vi "PH_gentec_M-Link.set Wavelength.vi"(0 "i ref in":refnum<vi>, 2 "VISA resource in":refnum<visa-resource-name>, 5 "error in":errorcluster) -> (11 "Timeout":bool, 13 "Data read":string[](array[string]), 14 "i ref out":refnum<vi>, 16 "VISA resource out":refnum<visa-resource-name>, 17 "Error":bool, 18 "Failure":bool, 19 "error out":errorcluster)   [LabVIEW 2014, in "PH_gentec_M-Link.lvlib"]
doc: "This VI writes wanted Settings to the Device and checks the result."
uses:
  PH_gentec_M-Link.lvlib
  instr.lib/Gentec-M-Link/gentec-M-Link - Driver.lvlib
  PH_Basics/PH_Powermeter_BaseClass/PH_Powermeter_BaseClass.lvlib
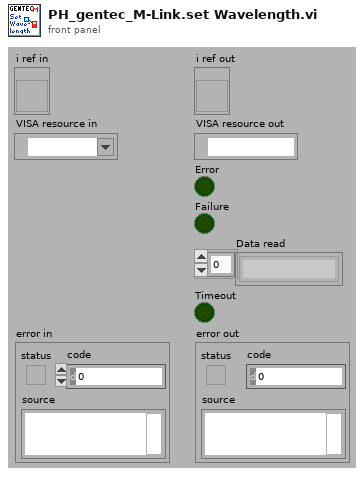
[diagram p1: front panel]
types:
  T1 = typedef "PH_Powermeter_BaseClass.lvlib/PH_Powermeter_BaseClass.i attribute.ctl" = cluster{"GUI References":T2, "Connection":T3, "Head Attributes":T5, "VISA resource":refnum<visa-resource-name>, "Energy":T6, "Service ID Energy":i32, "Wanted Settings":T7, "Current Settings":T7}
  T2 = typedef "PH_Powermeter_BaseClass.lvlib/PH_Powermeter_BaseClass.GUI Refs.ctl" = cluster{"Head Attributes":refnum<vi>, "Energy":refnum<vi>, "Connection":refnum<vi>, "VISA Resource":refnum<vi>, "Scaling Factor":refnum<vi>, "Range":refnum<vi>, "Wavelength":refnum<vi>, "Trigger Level":refnum<vi>, "Wanted Settings":refnum<vi>, "Current Settings":refnum<vi>}
  T3 = typedef "PH_Powermeter_BaseClass.lvlib/PH_Powermeter_BaseClass.Connection.ctl" = cluster{"failed checks":i8, "Timeout":bool, "Data read":string, "Failure":bool, "Error":bool, "State":T4}
  T4 = typedef "PH_Powermeter_BaseClass.lvlib/PH_Powermeter_BaseClass.State.ctl" = enum32{"off", "operating", "opened", "checked", "connected", "Sets to change", "running"}
  T5 = typedef "PH_Powermeter_BaseClass.lvlib/PH_Powermeter_BaseClass.Head Attributes.ctl" = cluster{"Instrument Type":string, "Head Version":string, "Head Name":string, "Serial Number":string, "Firmware":string, "Sensor Type":string, "MinimumRange":u32, "Maximum Range":u32, "Min Wavelength":i32, "Max Wavelength":i32}
  T6 = typedef "PH_Powermeter_BaseClass.lvlib/PH_Powermeter_BaseClass.Energy.ctl" = cluster{"current Value":dbl, "unscaled":dbl, "Scaling Factor":dbl}
  T7 = typedef "PH_Powermeter_BaseClass.lvlib/PH_gentec_BaseClass.Head Settings.ctl" = cluster{"Trigger Level":dbl, "Wavelength":u32, "Range":u32}
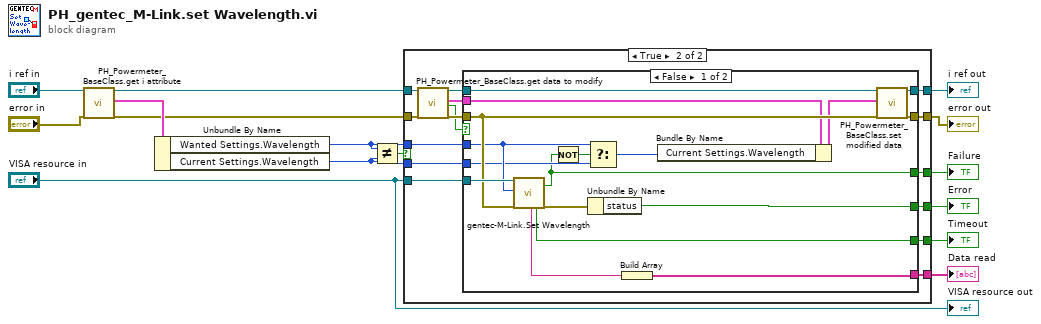
[diagram p0: block diagram]
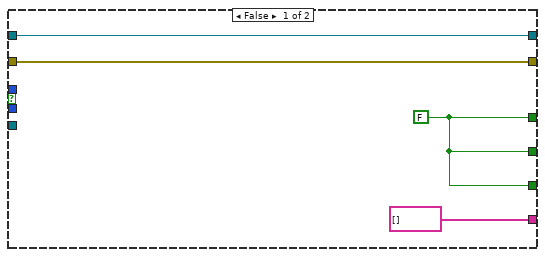
[diagram p2: hidden frame]
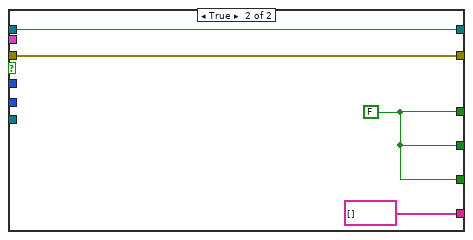
[diagram p3: hidden frame]
diagram:
  n1 = call "PH_Powermeter_BaseClass.get i attribute.vi"("i ref in"="i ref in", "error in (no error)"="error in") -> ("i ref out"=w9:refnum<vi>, "i attribute"=w12:T1, "error out"=w11:errorcluster)  [unwired: 15 in]
  n2 = Unbundle By Name(w12) -> ("Wanted Settings.Wavelength"=w13:u32, "Current Settings.Wavelength"=w1:u32)
  n3 = Not Equal?(x=w13, y=w1) -> (x != y?=w2:bool)
  n4 = case shown="True" w2 {
    tunnel: [w16 w34] -> w15
    tunnel: [w17 w33] -> w14
    tunnel: w13 -> [_ w32]
    tunnel: w11 -> [w16 w27]
    tunnel: w9 -> [w17 w26]
    tunnel: "VISA resource in" -> [_ w25]
    tunnel: [w19 w24] -> w6
    tunnel: [w19 w23] -> w5
    tunnel: [w19 w22] -> w4
    tunnel: [string[] [] w21] -> w3
    tunnel: w1 -> [_ w20]
    frame False {
      w19 = FALSE
    }
    frame True {
      n5 = call "PH_Powermeter_BaseClass.get data to modify.vi"("i ref in"=w26, "error in (no error)"=w27) -> ("i ref out"=w30:refnum<vi>, "i attribute"=w29:T1, "timed out"=w28:bool, "error out"=w31:errorcluster)  [unwired: 14 in]
      n6 = case shown="False" w28 {
        tunnel: w25 -> [w50 _]
        tunnel: [w47 w55] -> w33
        tunnel: [w46 w54] -> w34
        tunnel: w31 -> [w49 w54]
        tunnel: w30 -> [w51 w55]
        tunnel: w29 -> [w48 _]
        tunnel: w32 -> [w39 _]
        tunnel: [w44 w53] -> w24
        tunnel: [w36 w53] -> w23
        tunnel: [w43 w53] -> w22
        tunnel: [w42 string[] []] -> w21
        tunnel: w20 -> [w37 _]
        frame False {
          n7 = call "gentec-M-Link.Set Wavelength.vi"("VISA resource In"=w50, "Lambda"=w39, "error in (no error)"=w49) -> ("Data Read"=w41:string, "Error"=w36:bool, "Read Timeout"=w43:bool, "error out"=w38:errorcluster)  [unwired: 8 in, 5 out]
          n8 = Not(x=w36) -> (.not. x?=w35:bool)
          n9 = Select(t=w39, s=w35, f=w37) -> (s? t:f=w40:u32)
          n10 = Unbundle By Name(w38) -> ("status"=w44:bool)
          n11 = Build Array(w41) -> (w42:string[])
          n12 = Bundle By Name(cluster=w48, "Current Settings.Wavelength"=w40) -> (w45:T1)
          n13 = call "PH_Powermeter_BaseClass.set modified data.vi"("i ref in"=w51, "i attribute"=w45, "error in (no error)"=w49) -> ("i ref out"=w47:refnum<vi>, "error out"=w46:errorcluster)  [unwired: 15 in]
        }
        frame True {
          w53 = FALSE
        }
      }
    }
  }
  "error out" <- w15
  "i ref out" <- w14
  "Error" <- w6
  "Failure" <- w5
  "Timeout" <- w4
  "Data read" <- w3
  "VISA resource out" <- "VISA resource in"
